vi "LaserLineDetection_Intensity_LeastSquare.vi"(0 "Image In":T1, 1 "I_AVERAGEarray In":u8[](array[numeric]), 2 "Loop Count":i32, 5 "Xarray In":i32[](array[numeric]), 7 "Yarray In":i32[](array[numeric]), 9 "INTENSITYarray In":u8[](array[numeric]), 11 "error in (no error)":errorcluster, 12 "tolerance (residue)":dbl) -> (3 "I_AVERAGEarray Out":u8[](array[numeric]), 4 "Image Out":T1, 6 "slope":dbl, 8 "intercept":dbl, 10 "INTENSITYarray Out":u8[](array[numeric]), 13 "Yarray Out":i32[](array[numeric]), 14 "Least Square Accepted":bool, 15 "error out":errorcluster)   [LabVIEW 2013]
uses:
  <vilib>/vision/Image Controls.llb/IMAQ Image.ctl
  <vilib>/Analysis/6fits.llb/Curve Fitting Criteria.ctl
  <vilib>/Analysis/NI_AALPro.lvlib
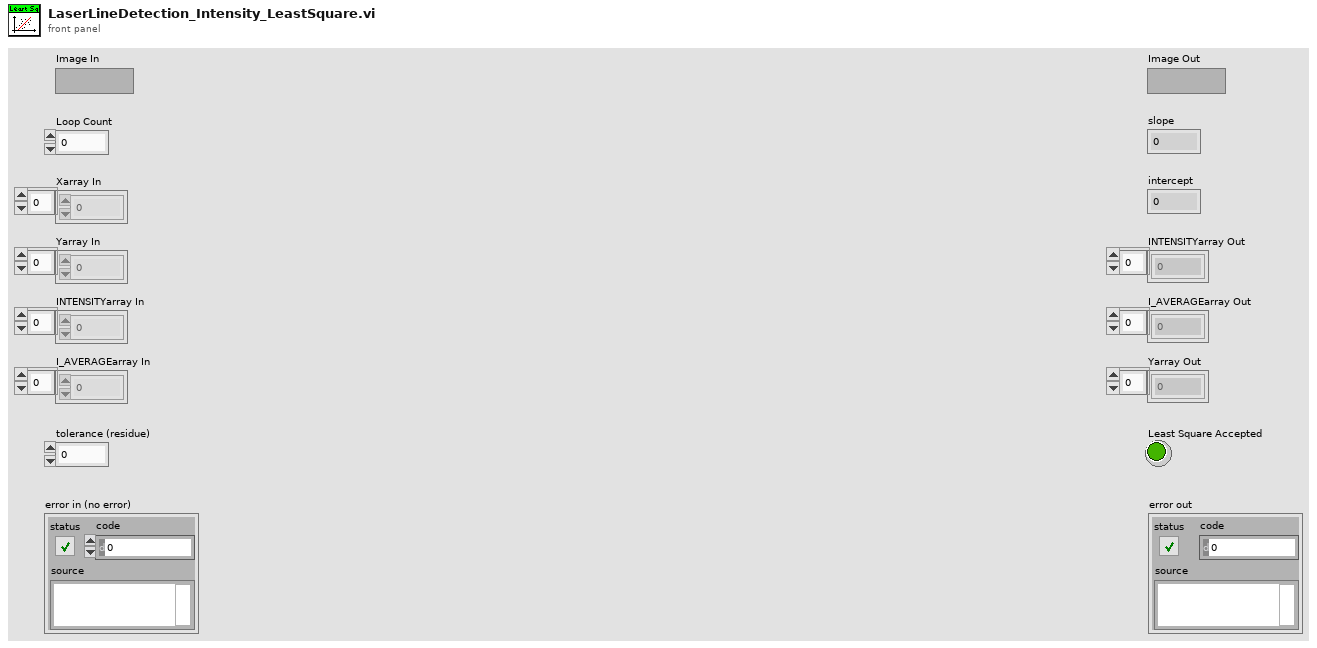
[diagram p1: front panel]
types:
  T1 = typedef "IMAQ Image.ctl" = refnum<image>
  T2 = cluster{"slope min":dbl, "slope max":dbl, "intercept min":dbl, "intercept max":dbl}
  T3 = typedef "NI_AALPro.lvlib/Curve Fitting Criteria.ctl" = u16
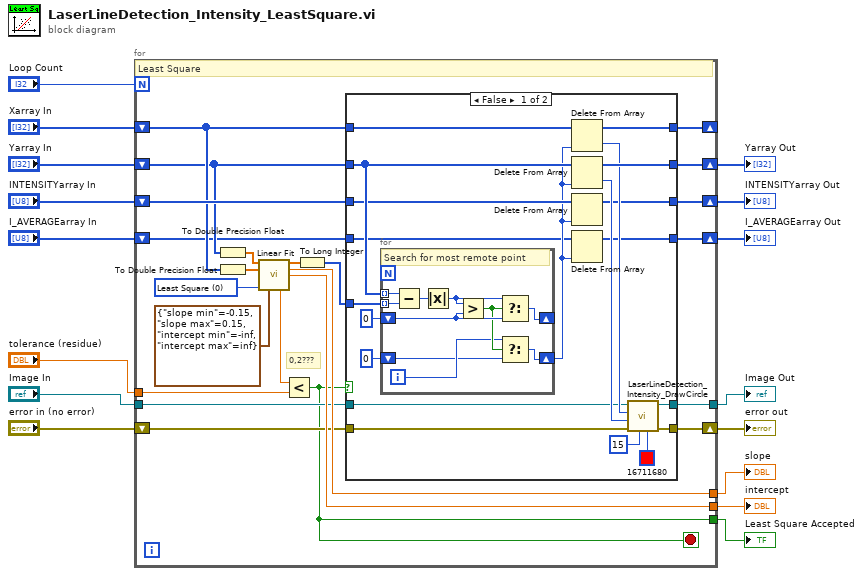
[diagram p0: block diagram]
diagram:
  n1 = for {
    N: "Loop Count" -> [_]
    tunnel: [w38] -> w11
    tunnel: [w37] -> w10
    shift-right: [w35] -> w1
    shift-left: "Yarray In" -> [w22]
    shift-right: [w34] -> _
    shift-left: "Xarray In" -> [w23]
    tunnel: "Image In" -> [w32]
    tunnel: [w31] -> w7
    shift-right: [w29] -> w9
    shift-left: "error in (no error)" -> [w30]
    tunnel: [w26] -> w12
    shift-right: [w24] -> w4
    shift-left: "INTENSITYarray In" -> [w25]
    tunnel: "tolerance (residue)" -> [w19]
    shift-right: [w17] -> w2
    shift-left: "I_AVERAGEarray In" -> [w18]
    stop <- w26 stop-if-true
    w39 = T3 0 items=["Least Square", "Least Absolute Residual", "Bisquare"] ("method")
    # "0,2???"
    # "Least Square"
    n2 = To Double Precision Float(number=w22) -> (double precision float=w21:dbl[])
    n3 = To Double Precision Float(number=w23) -> (double precision float=w20:dbl[])
    n4 = call <vilib>:"Linear Fit.vi"("Y"=w21, "X"=w20, "method"=w39, "parameter bounds"=T2 {"slope min"=-0.15, "slope max"=0.15, "intercept min"=-inf, "intercept max"=inf}) -> ("Best Linear Fit"=w27:dbl[], "slope"=w37:dbl, "intercept"=w38:dbl, "residue"=w36:dbl)  [unwired: 7 in, 1 out]
    n5 = Less?(x=w36, y=w19) -> (x < y?=w26:bool)
    n6 = To Long Integer(number=w27) -> (32bit integer=w33:i32[])
    n7 = case shown="False" w26 {
      tunnel: w22 -> [w56 w74]
      tunnel: w33 -> [w59 _]
      tunnel: [w55 w74] -> w35
      tunnel: w23 -> [w54 w75]
      tunnel: [w53 w75] -> w34
      tunnel: w32 -> [w48 w73]
      tunnel: [w47 w73] -> w31
      tunnel: w30 -> [w46 w72]
      tunnel: [w45 w72] -> w29
      tunnel: w25 -> [w44 w71]
      tunnel: [w43 w71] -> w24
      tunnel: w18 -> [w41 w70]
      tunnel: [w40 w70] -> w17
      frame False {
        n8 = for {
          tunnel: w56 -> [w69] mode=indexing
          tunnel: w59 -> [w68] mode=indexing
          shift-right: [w66] -> _
          shift-left: 0 ("y") -> [w65]
          shift-right: [w60] -> w42
          shift-left: 0 ("f") -> [w61]
          i -> [w62]
          # "Search for most remote point"
          n9 = Subtract(x=w69, y=w68) -> (x-y=w67:i32)
          n10 = Absolute Value(x=w67) -> (abs(x)=w64:i32)
          n11 = Greater?(x=w64, y=w65) -> (0:w63:bool)
          n12 = Select(t=w64, s=w63, f=w65) -> (s? t:f=w66:i32)
          n13 = Select(t=w62, s=w63, f=w61) -> (s? t:f=w60:i32)
        }
        n14 = Delete From Array(array=w54, index=w42) -> (deleted portion=w49:i32, array with subset deleted=w53:i32[])  [unwired: 1 in]
        n15 = Delete From Array(array=w56, index=w42) -> (deleted portion=w50:i32, array with subset deleted=w55:i32[])  [unwired: 1 in]
        n16 = Delete From Array(array=w44, index=w42) -> (array with subset deleted=w43:u8[])  [unwired: 1 in, 1 out]
        n17 = Delete From Array(array=w41, index=w42) -> (array with subset deleted=w40:u8[])  [unwired: 1 in, 1 out]
        n18 = call "LaserLineDetection_Intensity_DrawCircle.vi"("Color"=u32 16711680, "Radius"=15, "Error In"=w46, "Y_center"=w50, "X_center"=w49, "Image in"=w48) -> ("Error Out"=w45:errorcluster, "Image out"=w47:T1)  [unwired: 4 in]
      }
      frame True {
      }
    }
  }
  "Least Square Accepted" <- w12
  "intercept" <- w11
  "slope" <- w10
  "error out" <- w9
  "Image Out" <- w7
  "INTENSITYarray Out" <- w4
  "I_AVERAGEarray Out" <- w2
  "Yarray Out" <- w1
